vi "Run_Core.vi"(0 "String Operations in":refnum<class "String Functions.lvclass">, 11 "error in (no error)":errorcluster) -> (4 "String Operations out":refnum<class "String Functions.lvclass">, 6 "Return":variant, 15 "error out":errorcluster)   [LabVIEW 2019, in "String Functions.lvclass"]
uses:
  String Functions.lvclass
  String Functions.lvclass/String Functions.ctl
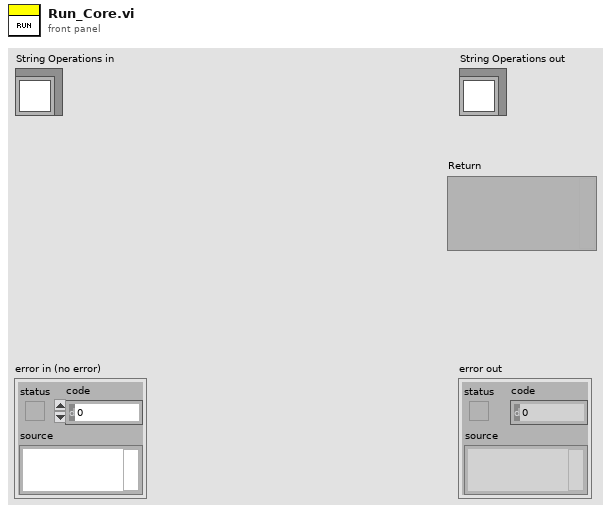
[diagram p1: front panel]
types:
  T1 = typedef "String Functions.lvclass/Function List.ctl" = enum16{"String Length", "Concatenate String", "String Subset", "Replace Substring", "To Upper Case", "To Lower Case", "Convert to String", "String to Number", "Random String", "String Reverse"}
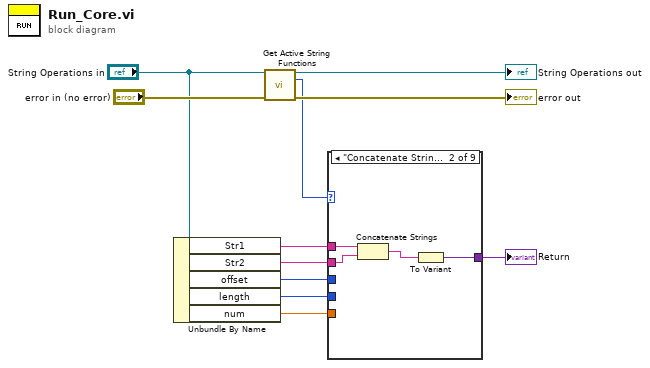
[diagram p0: block diagram]
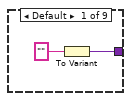
[diagram p2: hidden frame]
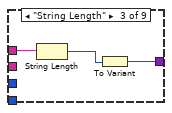
[diagram p3: hidden frame]
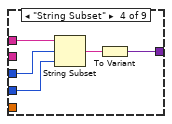
[diagram p4: hidden frame]
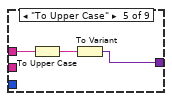
[diagram p5: hidden frame]
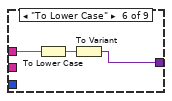
[diagram p6: hidden frame]
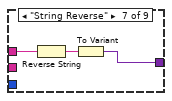
[diagram p7: hidden frame]
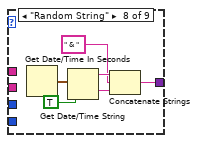
[diagram p8: hidden frame]
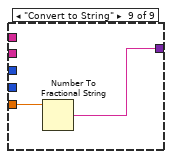
[diagram p9: hidden frame]
diagram:
  n1 = Unbundle By Name("String Operations in") -> ("Str1"=w11:string, "Str2"=w10:string, "offset"=w8:i32, "length"=w7:i32, "num"=w1:dbl)
  n2 = call "Get Active String Functions.vi"("String Functions in"="String Operations in", "error in (no error)"="error in (no error)") -> ("String Functions out"=→"String Operations out":refnum<class "String Functions.lvclass">, "Function List"=w2:T1, "error out"=→"error out":errorcluster)  [unwired: 11 in]
  n3 = case shown="\"Concatenate String\"" w2 {
    tunnel: w11 -> [_ w17 w20 w25 w28 w31 w34 _ _]
    tunnel: w10 -> [_ w16 _ _ _ _ _ _ _]
    tunnel: [w12 w14 w18 w21 w26 w29 w32 w35 w41] -> w9
    tunnel: w8 -> [_ _ _ w24 _ _ _ _ _]
    tunnel: w7 -> [_ _ _ w23 _ _ _ _ _]
    tunnel: w1 -> [_ _ _ _ _ _ _ _ w42]
    frame Default {
      n4 = To Variant(anything="") -> (Variant=w12:variant)
    }
    frame "Concatenate String" {
      n5 = Concatenate Strings(w17, w16) -> (w15:string)
      n6 = To Variant(anything=w15) -> (Variant=w14:variant)
    }
    frame "String Length" {
      n7 = String Length(string=w20) -> (length=w19:i32)
      n8 = To Variant(anything=w19) -> (Variant=w18:variant)
    }
    frame "String Subset" {
      n9 = String Subset(string=w25, offset (0)=w24, length (rest)=w23) -> (substring=w22:string)
      n10 = To Variant(anything=w22) -> (Variant=w21:variant)
    }
    frame "To Upper Case" {
      n11 = To Upper Case(1:w28) -> (0:w27:string)
      n12 = To Variant(anything=w27) -> (Variant=w26:variant)
    }
    frame "To Lower Case" {
      n13 = To Lower Case(string=w31) -> (all lower case string=w30:string)
      n14 = To Variant(anything=w30) -> (Variant=w29:variant)
    }
    frame "String Reverse" {
      n15 = Reverse String(1:w34) -> (0:w33:string)
      n16 = To Variant(anything=w33) -> (Variant=w32:variant)
    }
    frame "Random String" {
      n17 = Get Date/Time In Seconds() -> (seconds since 1Jan1904=w40:timestamp)
      n18 = Get Date/Time String(seconds (now)=w40, want seconds? (F)=TRUE) -> (date string=w39:string, time string=w38:string)  [unwired: 1 in]
      n19 = Concatenate Strings(w39, " & " ("string"), w38) -> (w35:string)
    }
    frame "Convert to String" {
      n20 = Number To Fractional String(number=w42) -> (F-format string=w41:string)  [unwired: 3 in]
    }
  }
  "Return" <- w9
